vi "tareaRGB.vi"() -> ()   [LabVIEW 2020]
panel:
  out "0GB 2":picture
  out "R0B 2":picture
  out "255GB 3":picture
  out "R255G 2":picture
  out "R255G":picture
  out "255GB":picture
  out "RG255":picture
  out "R0B":picture
  out "0GB":picture
  out "RG0":picture
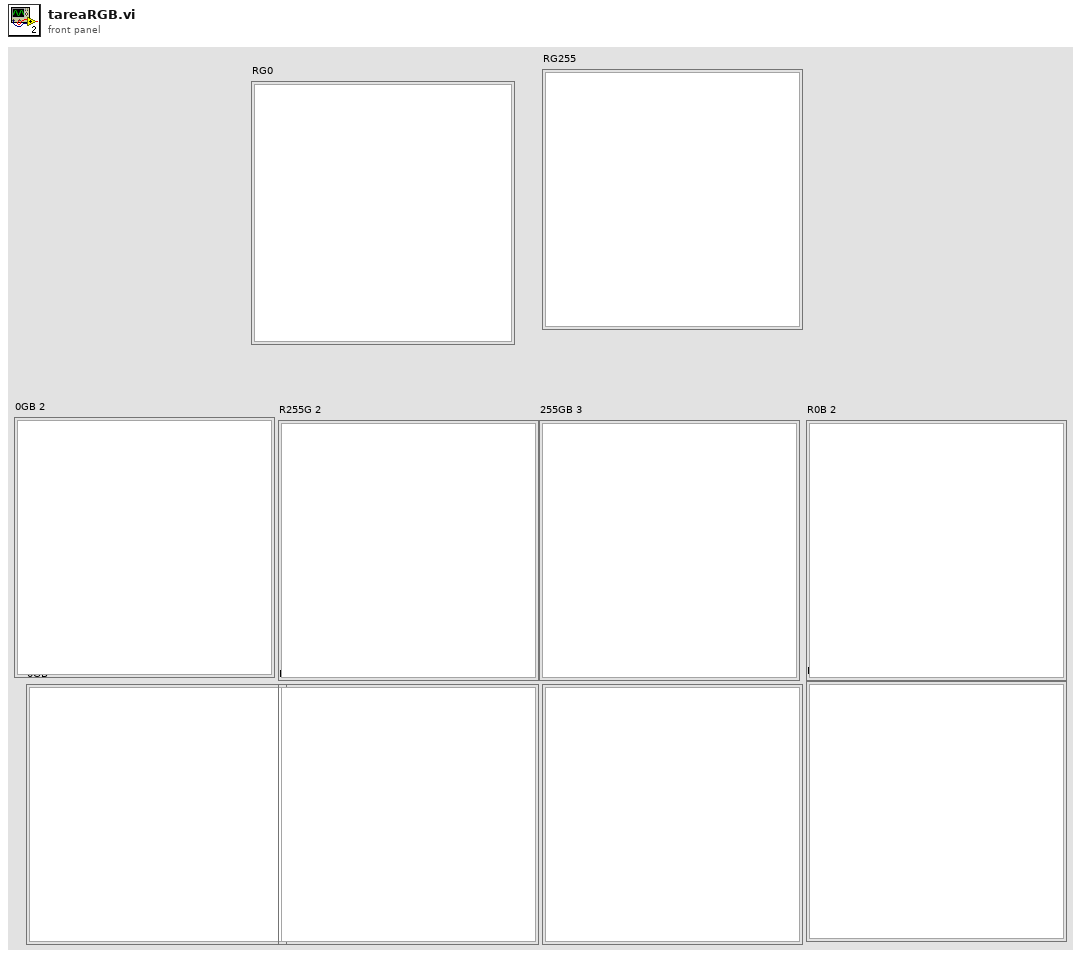
[diagram p1: front panel]
types:
  T1 = typedef "imagedata.ctl" = cluster{"image type":i32, "image depth":i32, "image":u8[], "mask":u8[], "colors":u32[], "Rectangle":cluster{"left":i16, "top":i16, "right":i16, "bottom":i16}}
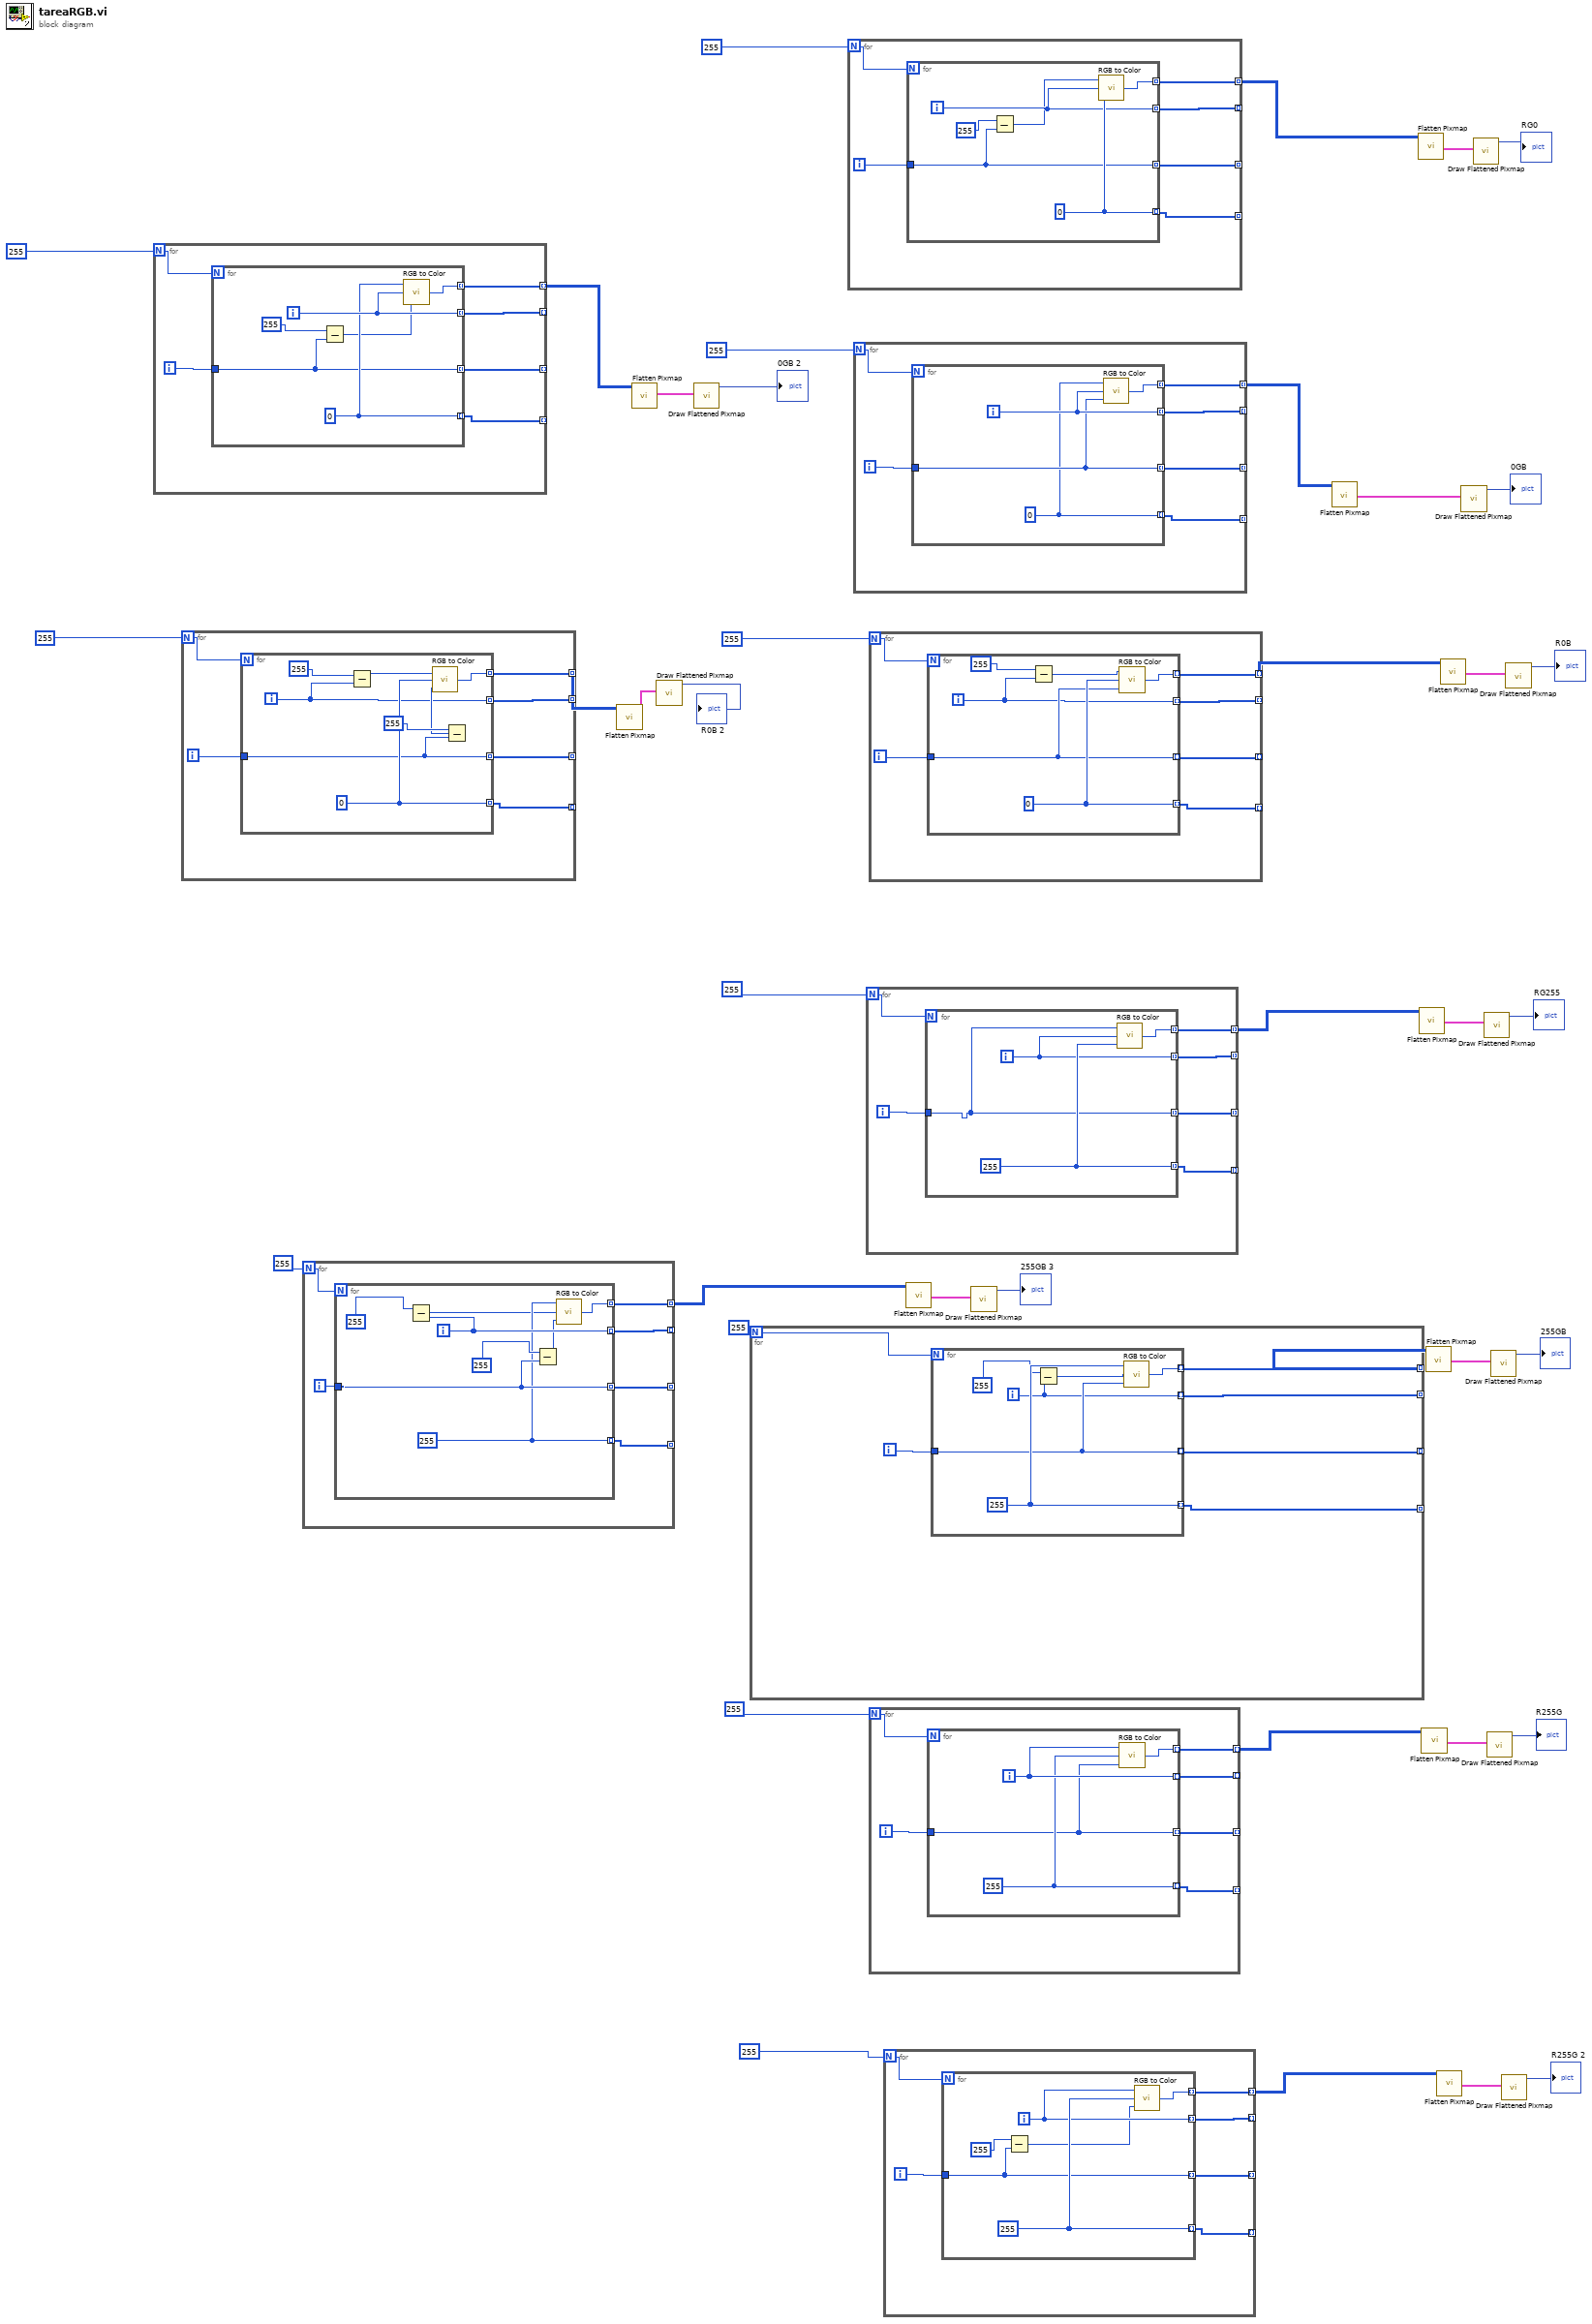
[diagram p0: block diagram]
diagram:
  n1 = for {
    N: 255 -> [w42]
    tunnel: [w46] -> _ mode=indexing
    tunnel: [w44] -> _ mode=indexing
    tunnel: [w43] -> _ mode=indexing
    tunnel: [w41] -> w1 mode=indexing
    i -> [w45]
    n2 = for {
      N: w42 -> [_]
      tunnel: [w51] -> w46 mode=indexing
      tunnel: w45 -> [w47]
      tunnel: [w47] -> w44 mode=indexing
      tunnel: [w50] -> w43 mode=indexing
      tunnel: [w52] -> w41 mode=indexing
      i -> [w51]
      w50 = 0
      n3 = Subtract(x=255, y=w47) -> (x-y=w48:i32)
      n4 = call <vilib>:"RGB to Color.vi"("B"=w48, "G"=w51, "R"=w50) -> ("Color"=w52:u32)
    }
  }
  n5 = for {
    N: 255 -> [w54]
    tunnel: [w58] -> _ mode=indexing
    tunnel: [w56] -> _ mode=indexing
    tunnel: [w55] -> _ mode=indexing
    tunnel: [w53] -> w5 mode=indexing
    i -> [w57]
    n6 = for {
      N: w54 -> [_]
      tunnel: [w60] -> w58 mode=indexing
      tunnel: w57 -> [w59]
      tunnel: [w59] -> w56 mode=indexing
      tunnel: [w65] -> w55 mode=indexing
      tunnel: [w66] -> w53 mode=indexing
      i -> [w60]
      w65 = 0
      n7 = Subtract(x=255, y=w60) -> (x-y=w63:i32)
      n8 = Subtract(x=255, y=w59) -> (x-y=w61:i32)
      n9 = call <vilib>:"RGB to Color.vi"("B"=w61, "G"=w65, "R"=w63) -> ("Color"=w66:u32)
    }
  }
  n10 = for {
    N: 255 -> [w68]
    tunnel: [w72] -> _ mode=indexing
    tunnel: [w70] -> _ mode=indexing
    tunnel: [w69] -> _ mode=indexing
    tunnel: [w67] -> w9 mode=indexing
    i -> [w71]
    n11 = for {
      N: w68 -> [_]
      tunnel: [w78] -> w72 mode=indexing
      tunnel: w71 -> [w75]
      tunnel: [w75] -> w70 mode=indexing
      tunnel: [w74] -> w69 mode=indexing
      tunnel: [w80] -> w67 mode=indexing
      i -> [w78]
      w74 = 255
      n12 = Subtract(x=255, y=w78) -> (x-y=w73:i32)
      n13 = Subtract(x=255, y=w75) -> (x-y=w76:i32)
      n14 = call <vilib>:"RGB to Color.vi"("B"=w76, "G"=w73, "R"=w74) -> ("Color"=w80:u32)
    }
  }
  n15 = call <vilib>:"Flatten Pixmap.vi"("24-bit pixmap"=w5) -> ("image data"=w8:T1)  [unwired: 10 in]
  n16 = call <vilib>:"Flatten Pixmap.vi"("24-bit pixmap"=w1) -> ("image data"=w3:T1)  [unwired: 10 in]
  n17 = call <vilib>:"Draw Flattened Pixmap.vi"("image data"=w8) -> ("new picture"=→"R0B 2":picture)  [unwired: 8 in]
  n18 = call <vilib>:"Draw Flattened Pixmap.vi"("image data"=w3) -> ("new picture"=→"0GB 2":picture)  [unwired: 8 in]
  n19 = for {
    N: 255 -> [w82]
    tunnel: [w86] -> _ mode=indexing
    tunnel: [w84] -> _ mode=indexing
    tunnel: [w83] -> _ mode=indexing
    tunnel: [w81] -> w21 mode=indexing
    i -> [w85]
    n20 = for {
      N: w82 -> [_]
      tunnel: [w87] -> w86 mode=indexing
      tunnel: w85 -> [w90]
      tunnel: [w90] -> w84 mode=indexing
      tunnel: [w91] -> w83 mode=indexing
      tunnel: [w92] -> w81 mode=indexing
      i -> [w87]
      w91 = 255
      n21 = Subtract(x=255, y=w87) -> (x-y=w88:i32)
      n22 = call <vilib>:"RGB to Color.vi"("B"=w90, "G"=w88, "R"=w91) -> ("Color"=w92:u32)
    }
  }
  n23 = for {
    N: 255 -> [w94]
    tunnel: [w98] -> _ mode=indexing
    tunnel: [w96] -> _ mode=indexing
    tunnel: [w95] -> _ mode=indexing
    tunnel: [w93] -> w29 mode=indexing
    i -> [w97]
    n24 = for {
      N: w94 -> [_]
      tunnel: [w102] -> w98 mode=indexing
      tunnel: w97 -> [w99]
      tunnel: [w99] -> w96 mode=indexing
      tunnel: [w104] -> w95 mode=indexing
      tunnel: [w103] -> w93 mode=indexing
      i -> [w102]
      w104 = 0
      n25 = Subtract(x=255, y=w99) -> (x-y=w101:i32)
      n26 = call <vilib>:"RGB to Color.vi"("B"=w104, "G"=w102, "R"=w101) -> ("Color"=w103:u32)
    }
  }
  n27 = for {
    N: 255 -> [w106]
    tunnel: [w110] -> _ mode=indexing
    tunnel: [w108] -> _ mode=indexing
    tunnel: [w107] -> _ mode=indexing
    tunnel: [w105] -> w32 mode=indexing
    i -> [w109]
    n28 = for {
      N: w106 -> [_]
      tunnel: [w113] -> w110 mode=indexing
      tunnel: w109 -> [w112]
      tunnel: [w112] -> w108 mode=indexing
      tunnel: [w111] -> w107 mode=indexing
      tunnel: [w114] -> w105 mode=indexing
      i -> [w113]
      w111 = 0
      n29 = call <vilib>:"RGB to Color.vi"("B"=w112, "G"=w113, "R"=w111) -> ("Color"=w114:u32)
    }
  }
  n30 = for {
    N: 255 -> [w116]
    tunnel: [w120] -> _ mode=indexing
    tunnel: [w118] -> _ mode=indexing
    tunnel: [w117] -> _ mode=indexing
    tunnel: [w115] -> w25 mode=indexing
    i -> [w119]
    n31 = for {
      N: w116 -> [_]
      tunnel: [w121] -> w120 mode=indexing
      tunnel: w119 -> [w122]
      tunnel: [w122] -> w118 mode=indexing
      tunnel: [w123] -> w117 mode=indexing
      tunnel: [w124] -> w115 mode=indexing
      i -> [w121]
      w123 = 255
      n32 = call <vilib>:"RGB to Color.vi"("B"=w123, "G"=w121, "R"=w122) -> ("Color"=w124:u32)
    }
  }
  n33 = for {
    N: 255 -> [w126]
    tunnel: [w130] -> _ mode=indexing
    tunnel: [w128] -> _ mode=indexing
    tunnel: [w127] -> _ mode=indexing
    tunnel: [w125] -> w30 mode=indexing
    i -> [w129]
    n34 = for {
      N: w126 -> [_]
      tunnel: [w131] -> w130 mode=indexing
      tunnel: w129 -> [w132]
      tunnel: [w132] -> w128 mode=indexing
      tunnel: [w135] -> w127 mode=indexing
      tunnel: [w136] -> w125 mode=indexing
      i -> [w131]
      w135 = 0
      n35 = Subtract(x=255, y=w131) -> (x-y=w133:i32)
      n36 = call <vilib>:"RGB to Color.vi"("B"=w132, "G"=w135, "R"=w133) -> ("Color"=w136:u32)
    }
  }
  n37 = for {
    N: 255 -> [w138]
    tunnel: [w142] -> _ mode=indexing
    tunnel: [w140] -> _ mode=indexing
    tunnel: [w139] -> _ mode=indexing
    tunnel: [w137] -> w17 mode=indexing
    i -> [w141]
    n38 = for {
      N: w138 -> [_]
      tunnel: [w145] -> w142 mode=indexing
      tunnel: w141 -> [w143]
      tunnel: [w143] -> w140 mode=indexing
      tunnel: [w144] -> w139 mode=indexing
      tunnel: [w146] -> w137 mode=indexing
      i -> [w145]
      w144 = 255
      n39 = call <vilib>:"RGB to Color.vi"("B"=w143, "G"=w144, "R"=w145) -> ("Color"=w146:u32)
    }
  }
  n40 = for {
    N: 255 -> [w148]
    tunnel: [w152] -> _ mode=indexing
    tunnel: [w150] -> _ mode=indexing
    tunnel: [w149] -> _ mode=indexing
    tunnel: [w147] -> w13 mode=indexing
    i -> [w151]
    n41 = for {
      N: w148 -> [_]
      tunnel: [w156] -> w152 mode=indexing
      tunnel: w151 -> [w153]
      tunnel: [w153] -> w150 mode=indexing
      tunnel: [w157] -> w149 mode=indexing
      tunnel: [w158] -> w147 mode=indexing
      i -> [w156]
      w157 = 255
      n42 = Subtract(x=255, y=w153) -> (x-y=w154:i32)
      n43 = call <vilib>:"RGB to Color.vi"("B"=w154, "G"=w157, "R"=w156) -> ("Color"=w158:u32)
    }
  }
  n44 = call <vilib>:"Flatten Pixmap.vi"("24-bit pixmap"=w9) -> ("image data"=w11:T1)  [unwired: 10 in]
  n45 = call <vilib>:"Draw Flattened Pixmap.vi"("image data"=w11) -> ("new picture"=→"255GB 3":picture)  [unwired: 8 in]
  n46 = call <vilib>:"Flatten Pixmap.vi"("24-bit pixmap"=w32) -> ("image data"=w36:T1)  [unwired: 10 in]
  n47 = call <vilib>:"Flatten Pixmap.vi"("24-bit pixmap"=w29) -> ("image data"=w39:T1)  [unwired: 10 in]
  n48 = call <vilib>:"Flatten Pixmap.vi"("24-bit pixmap"=w25) -> ("image data"=w27:T1)  [unwired: 10 in]
  n49 = call <vilib>:"Flatten Pixmap.vi"("24-bit pixmap"=w17) -> ("image data"=w19:T1)  [unwired: 10 in]
  n50 = call <vilib>:"Flatten Pixmap.vi"("24-bit pixmap"=w21) -> ("image data"=w23:T1)  [unwired: 10 in]
  n51 = call <vilib>:"Flatten Pixmap.vi"("24-bit pixmap"=w13) -> ("image data"=w15:T1)  [unwired: 10 in]
  n52 = call <vilib>:"Flatten Pixmap.vi"("24-bit pixmap"=w30) -> ("image data"=w35:T1)  [unwired: 10 in]
  n53 = call <vilib>:"Draw Flattened Pixmap.vi"("image data"=w36) -> ("new picture"=→"0GB":picture)  [unwired: 8 in]
  n54 = call <vilib>:"Draw Flattened Pixmap.vi"("image data"=w39) -> ("new picture"=→"RG0":picture)  [unwired: 8 in]
  n55 = call <vilib>:"Draw Flattened Pixmap.vi"("image data"=w27) -> ("new picture"=→"RG255":picture)  [unwired: 8 in]
  n56 = call <vilib>:"Draw Flattened Pixmap.vi"("image data"=w19) -> ("new picture"=→"R255G":picture)  [unwired: 8 in]
  n57 = call <vilib>:"Draw Flattened Pixmap.vi"("image data"=w23) -> ("new picture"=→"255GB":picture)  [unwired: 8 in]
  n58 = call <vilib>:"Draw Flattened Pixmap.vi"("image data"=w15) -> ("new picture"=→"R255G 2":picture)  [unwired: 8 in]
  n59 = call <vilib>:"Draw Flattened Pixmap.vi"("image data"=w35) -> ("new picture"=→"R0B":picture)  [unwired: 8 in]
